vi "Set Target.vi"(8 "error in (no error)":errorcluster, 9 "Target Rate (T/min)":dbl, 10 "Target Field (T)":dbl, 11 "Instrument.1820 in":refnum<class "Instrument.OxfordVRM.lvclass">) -> (0 "error out":errorcluster, 2 "Response":string, 3 "Instrument.1820 in":refnum<class "Instrument.OxfordVRM.lvclass">)   [LabVIEW 2016, in "Instrument.OxfordVRM.lvclass"]
uses:
  Instrument.OxfordVRM.lvclass
  Typedefs/Targets.ctl
  Typedefs/Instrument.Oxford1820.Commands-enum.ctl
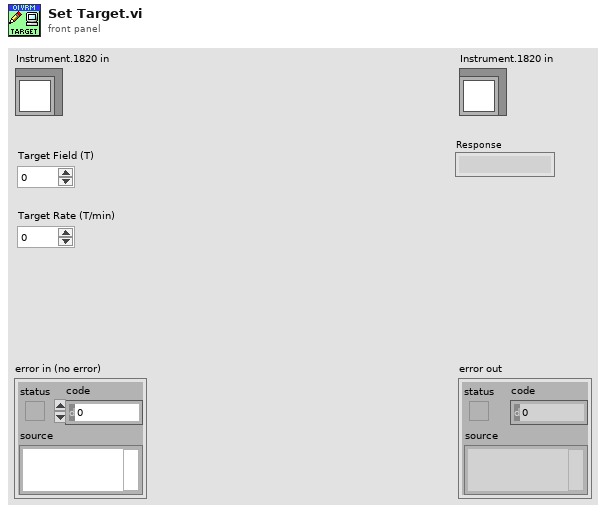
[diagram p1: front panel]
types:
  T1 = typedef "Instrument.OxfordVRM.lvclass/Instrument.Oxford1820.Commands-enum.ctl" = enum16{"setAction", "setTarget", "setSwitchHeat", "setLambda", "setFillMode", "setNeedleValve", "setMagnetField", "getStatus", "getTarget", "getSwitchHeat", "getPSUField", "newcommand", "getMagnetField"}
  T2 = typedef "Instrument.OxfordVRM.lvclass/Targets.ctl" = cluster{"Field (T)":dbl, "Field Rate (T/min)":dbl}
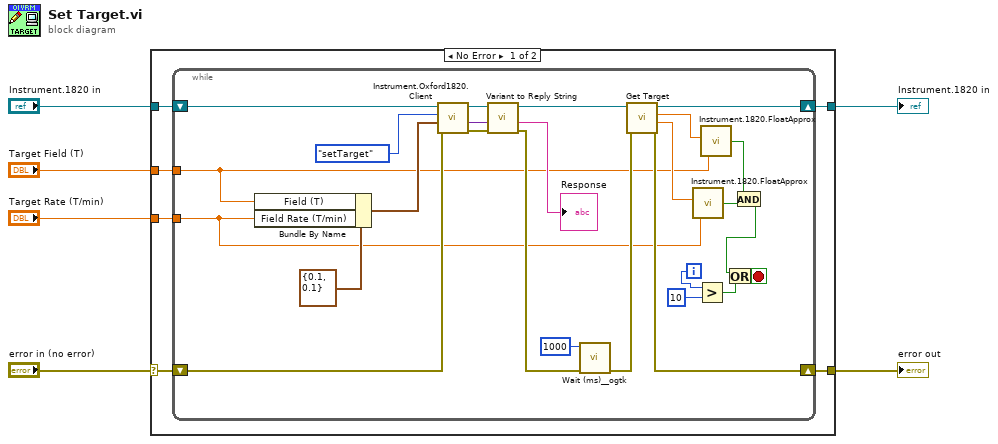
[diagram p0: block diagram]
diagram:
  n1 = case shown="No Error" "error in (no error)" {
    selector: "error in (no error)" -> [w9 w40]
    tunnel: "Target Rate (T/min)" -> [w12 _]
    tunnel: [w7 w40] -> w5
    tunnel: "Target Field (T)" -> [w11 _]
    tunnel: "Instrument.1820 in" -> [w10 w39]
    tunnel: [w8 w39] -> w1
    frame No Error {
      n2 = while {
        tunnel: w12 -> [w17]
        tunnel: w11 -> [w16]
        shift-right: [w34] -> w8
        shift-left: w10 -> [w29]
        shift-right: [w33] -> w7
        shift-left: w9 -> [w35]
        i -> [w25]
        stop <- w26 stop-if-true
        n3 = Bundle By Name(cluster=T2 {"Field (T)"=0.1, "Field Rate (T/min)"=0.1} ("Mercury Targets"), "Field (T)"=w16, "Field Rate (T/min)"=w17) -> (w36:T2)
        n4 = call "Instrument.Oxford1820.Client.vi"("error in (no error)"=w35, "Data"=w36, "Commands"=Instrument.Oxford1820.Commands-enum."setTarget", "Instrument.1820 in"=w29) -> ("error out"=w23:errorcluster, "Data out"=w24:variant, "Instrument.1820 out"=w22:refnum<class "Instrument.OxfordVRM.lvclass">)  [unwired: 5 in]
        n5 = call "Variant to Reply String.vi"("error in (no error)"=w23, "Data"=w24, "Instrument.1820 in"=w22) -> ("error out"=w20:errorcluster, "Reply"=→"Response":string, "Instrument.1820 out"=w21:refnum<class "Instrument.OxfordVRM.lvclass">)  [unwired: 6 in]
        n6 = call <userlib>:"Wait (ms)__ogtk.vi"("error in (no error)"=w20, "milliseconds to wait"=u32 1000) -> ("error out"=w32:errorcluster)  [unwired: 8 in, 1 out]
        n7 = call "Get Target.vi"("error in (no error)"=w32, "Instrument.1820 in"=w21) -> ("error out"=w33:errorcluster, "Target Field Rate (T/min)"=w18:dbl, "Target Field (T)"=w30:dbl, "Instrument.1820 in"=w34:refnum<class "Instrument.OxfordVRM.lvclass">)  [unwired: 6 in]
        n8 = call "Instrument.1820.FloatApprox.vi"("y"=w17, "x"=w18) -> ("x ~ y?"=w15:bool)  [unwired: 4 in]
        n9 = Greater?(x=w25, y=10) -> (0:w27:bool)
        n10 = call "Instrument.1820.FloatApprox.vi"("y"=w16, "x"=w30) -> ("x ~ y?"=w14:bool)  [unwired: 4 in]
        n11 = And(x=w14, y=w15) -> (x .and. y?=w13:bool)
        n12 = Or(x=w13, y=w27) -> (x .or. y?=w26:bool)
      }
    }
    frame Error {
    }
  }
  "Instrument.1820 in" <- w1
  "error out" <- w5
